vi "MaxAndMin.vi"() -> ()   [LabVIEW 2018]
panel:
  out "error out":errorcluster
  in  "Numbers":dbl[](array[numeric])=[0.0, -345.0, 245352.0, 23.0]
  out "Max and Min":cluster{"Max":dbl, "Min":dbl}
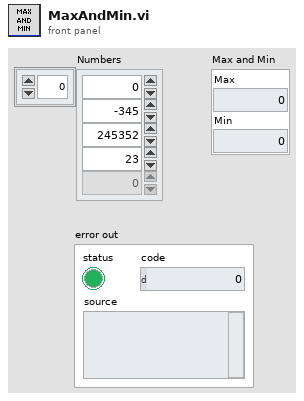
[diagram p1: front panel]
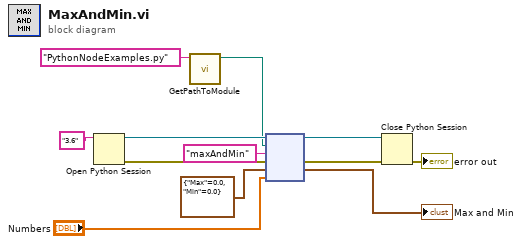
[diagram p0: block diagram]
diagram:
  n1 = Open Python Session(python version="3.6" ("Python version")) -> (session out=w12:refnum<k35>, error out=w5:errorcluster)  [unwired: 2 in]
  n2 = call "GetPathToModule.vi"("module name"="PythonNodeExamples.py") -> ("path to module"=w1:path)  [unwired: 10 in]
  n3 = node(w12, w1, "maxAndMin" ("function name"), w5, cluster{"Max":dbl, "Min":dbl} {"Max"=0.0, "Min"=0.0}, "Numbers") -> (w11:refnum<k35>, w4:errorcluster, →"Max and Min":cluster{"Max":dbl, "Min":dbl})  [unwired: 1 in, 2 out]
  n4 = Close Python Session(session in=w11, error in=w4) -> (11:→"error out":errorcluster)
